vi "parameter to Path_lvcicd.vi"(1 "String":string) -> (0 "Path":path)   [LabVIEW 2019]
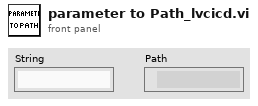
[diagram p1: front panel]
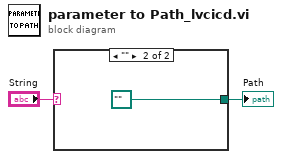
[diagram p0: block diagram]
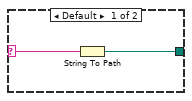
[diagram p2: hidden frame]
diagram:
  n1 = case shown="\"\"" "String" {
    selector: "String" -> [w4 _]
    tunnel: [w3 path ""] -> w1
    frame Default {
      n2 = String To Path(string=w4) -> (path=w3:path)
    }
    frame "" {
    }
  }
  "Path" <- w1
